vi "CustomGaugeFacade.vi"(0 "Data In":T4, 2 "Display State In":T2, 3 "Container State":T3) -> (6 "Data Out":T4, 7 "Display State Out":T2, 8 "Action":T1)   [LabVIEW 2012, in "CustomGauge.xctl"]
uses:
  CustomGauge.xctl
  CustomGaugeData.ctl
  <vilib>/_xctls/Container State.ctl
  CustomGaugeState.ctl
  <vilib>/_xctls/Action.ctl
  <vilib>/_xctls/XControlSupport.lvlib
panel:
  in  "Gauge":dbl(knob) scale=0.0..10.0
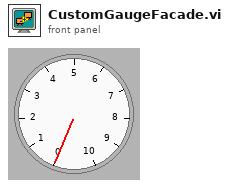
[diagram p1: front panel]
types:
  T1 = typedef "XControlSupport.lvlib/Action.ctl" = cluster{"Data Changed?":bool, "State Changed?":bool, "Action Name":string}
  T2 = typedef "CustomGauge.xctl/CustomGaugeState.ctl" = cluster{"Shared Variable Control":refnum<k21>}
  T3 = typedef "XControlSupport.lvlib/Container State.ctl" = cluster{"Indicator?":bool, "Run Mode?":bool, " Refnum":refnum<vi>}
  T4 = typedef "CustomGauge.xctl/CustomGaugeData.ctl" = dbl
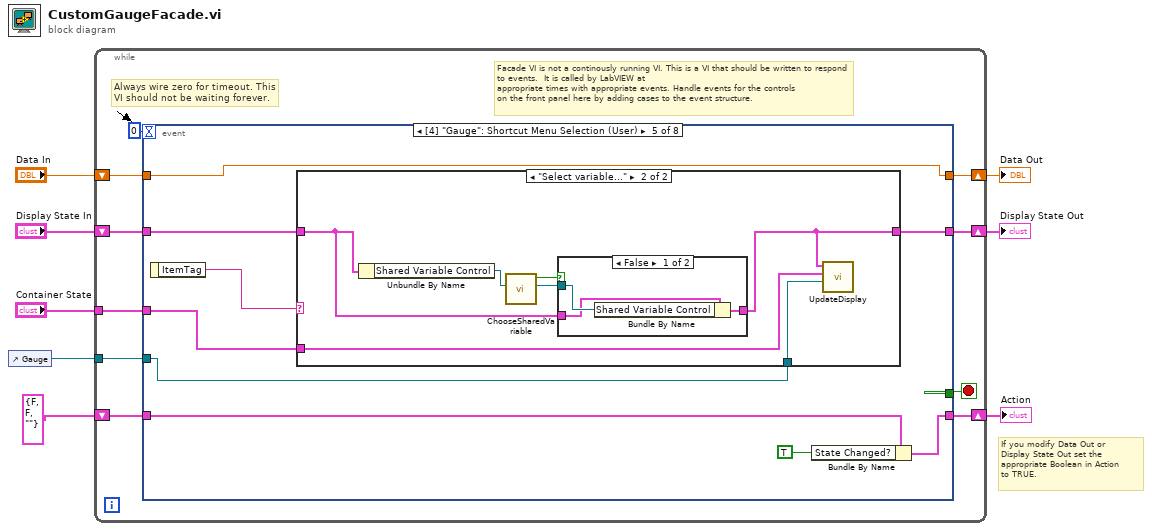
[diagram p0: block diagram]
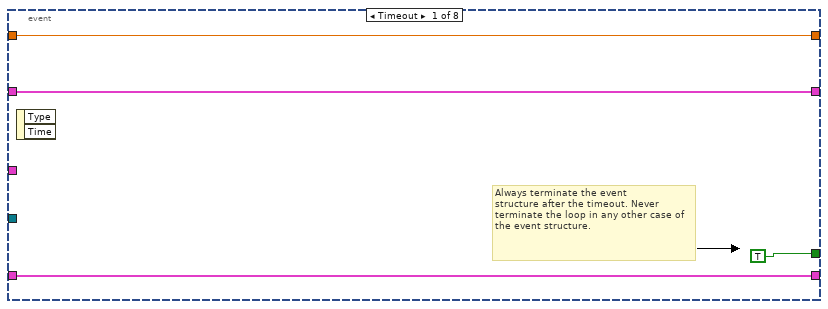
[diagram p2: hidden frame]
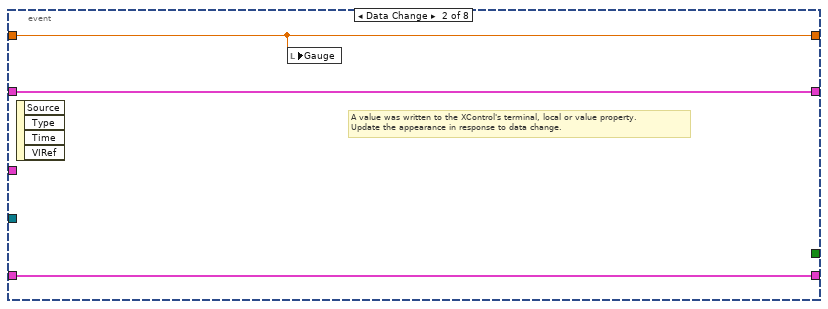
[diagram p3: hidden frame]
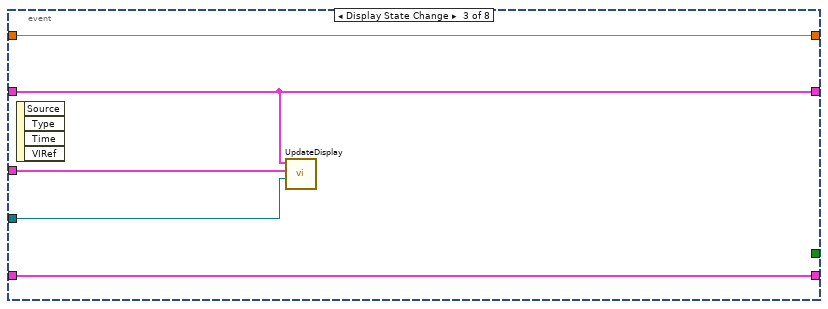
[diagram p4: hidden frame]
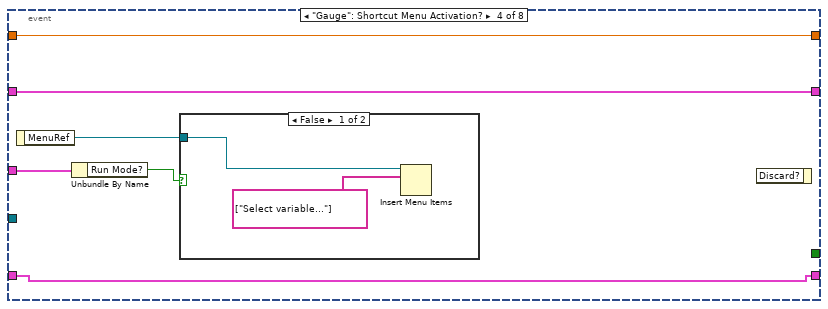
[diagram p5: hidden frame]
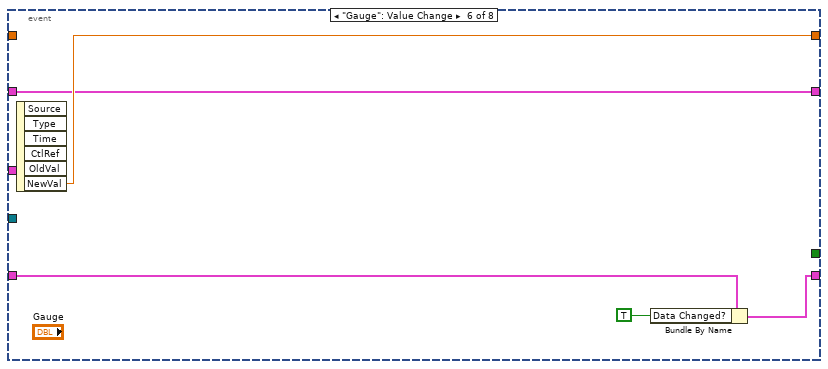
[diagram p9: hidden frame]
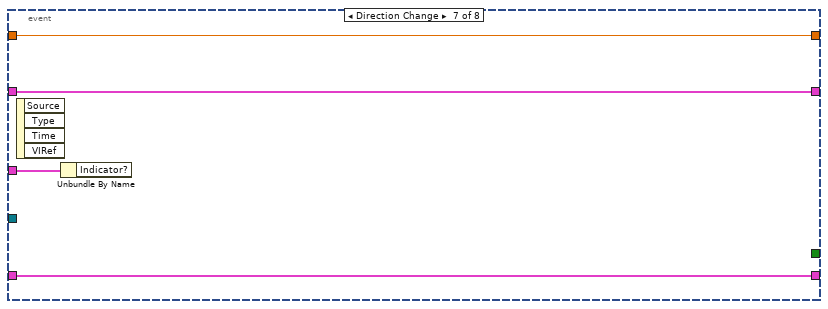
[diagram p10: hidden frame]
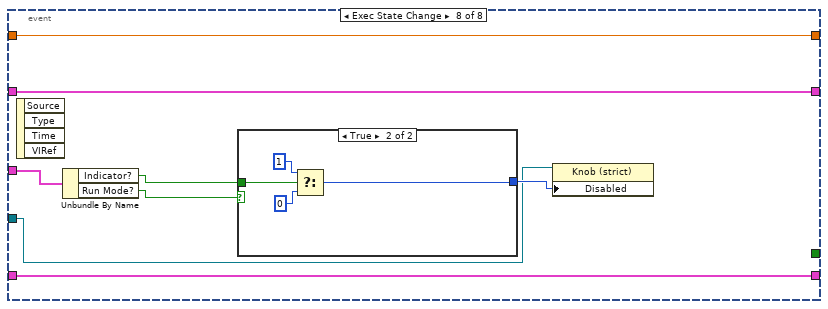
[diagram p11: hidden frame]
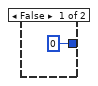
[diagram p12: hidden frame]
diagram:
  # "If you modify Data Out or\nDisplay State Out set the\nappropriate Boolean in Action\nto TRUE."
  n1 = control-ref of="Gauge"() -> (w1:refnum<vi>)
  n2 = while {
    shift-right: [w17] -> w5
    shift-left: "Display State In" -> [w18]
    tunnel: "Container State" -> [w14]
    shift-right: [w12] -> w8
    shift-left: "Data In" -> [w13]
    shift-right: [w10] -> w3
    shift-left: T1 {"Data Changed?"=FALSE, "State Changed?"=FALSE, "Action Name"=""} ("Action") -> [w11]
    tunnel: w1 -> [w9]
    stop <- w16 stop-if-true
    # "Facade VI is not a continously running VI. This is a VI that should be written to respond to events.  It is called by LabVIEW at\nappropriate times with appropriate events. Handle events for the controls\non the front panel here by adding cases to the event structure."
    # "Always wire zero for timeout. This\nVI should not be waiting forever."
    n3 = event shown="[4] \"Gauge\": Shortcut Menu Selection (User)" {
      selector: _ -> [_ _ _ _ _ _ _ _]
      dyn-events: _ -> [_ _ _ _ _ _ _ _]
      timeout: 0 -> [_ _ _ _ _ _ _ _]
      tunnel: w18 -> [w20 w25 w28 w35 w46 w63 w67 w75]
      tunnel: [w20 w25 w28 w35 w45 w63 w67 w75] -> w17
      tunnel: [TRUE _ _ _ _ _ _ _] -> w16
      tunnel: w14 -> [_ _ w27 w32 w40 _ w68 w76]
      tunnel: w13 -> [w19 w23 w30 w34 w44 _ w66 w74]
      tunnel: [w19 w23 w30 w34 w44 w64 w66 w74] -> w12
      tunnel: [w21 w24 w29 w33 w43 w62 w65 w73] -> w10
      tunnel: w11 -> [w21 w24 w29 w33 w42 w61 w65 w73]
      tunnel: w9 -> [_ _ w26 _ w39 _ _ w69]
      event Timeout {
        # "Always terminate the event\nstructure after the timeout. Never terminate the loop in any other case of the event structure."
        n4 = event-data() -> ()  [unwired: 1 in, 2 out]
      }
      event Data Change {
        # "A value was written to the XControl's terminal, local or value property.\nUpdate the appearance in response to data change."
        n5 = event-data() -> ()  [unwired: 1 in, 4 out]
        n6 = local write "Gauge"(w23) -> ()
      }
      event Display State Change {
        n7 = event-data() -> ()  [unwired: 1 in, 4 out]
        n8 = call "UpdateDisplay.vi"("Gauge"=w26, "Container State"=w27, "Display State In"=w28) -> ()  [unwired: 7 in, 1 out]
      }
      event "Gauge": Shortcut Menu Activation? {
        n9 = event-data() -> ("MenuRef"=w36:refnum<k9>)  [unwired: 1 in]
        n10 = Unbundle By Name(w32) -> ("Run Mode?"=w31:bool)
        n11 = case shown="False" w31 {
          tunnel: w36 -> [w38 _]
          frame False {
            n12 = Insert Menu Items(8:string[] ["Select variable..."] ("item names"), 9:w38) -> ()  [unwired: 4 in, 3 out]
          }
          frame True {
          }
        }
        n13 = event-data() -> ()  [unwired: 2 in, 1 out]
      }
      event "Gauge": Shortcut Menu Selection (User) {
        n14 = event-data() -> ("ItemTag"=w47:string)  [unwired: 1 in]
        n15 = case shown="\"Select variable...\"" w47 {
          tunnel: w46 -> [w48 w52]
          tunnel: [w48 w51] -> w45
          tunnel: w40 -> [_ w50]
          tunnel: w39 -> [_ w49]
          frame Default {
          }
          frame "Select variable..." {
            n16 = Unbundle By Name(w52) -> ("Shared Variable Control"=w53:refnum<k21>)
            n17 = call "ChooseSharedVariable.vi"("Select published shared variable to bind to..."=w53) -> ("Shared Variable"=w54:refnum<k21>, "Cancelled?"=w55:bool)  [unwired: 9 in]
            n18 = case shown="False" w55 {
              tunnel: w54 -> [w58 _]
              tunnel: [w57 w59] -> w51
              tunnel: w52 -> [w56 w59]
              frame False {
                n19 = Bundle By Name(cluster=w56, "Shared Variable Control"=w58) -> (w57:T2)
              }
              frame True {
              }
            }
            n20 = call "UpdateDisplay.vi"("Gauge"=w49, "Container State"=w50, "Display State In"=w51) -> ()  [unwired: 7 in, 1 out]
          }
        }
        n21 = Bundle By Name(cluster=w42, "State Changed?"=TRUE) -> (w43:T1)
      }
      event "Gauge": Value Change {
        n22 = event-data() -> ("NewVal"=w64:dbl)  [unwired: 1 in, 5 out]
        n23 = Bundle By Name(cluster=w61, "Data Changed?"=TRUE) -> (w62:T1)
      }
      event Direction Change {
        n24 = event-data() -> ()  [unwired: 1 in, 4 out]
        n25 = Unbundle By Name(w68) -> ()  [unwired: 1 out]
      }
      event Exec State Change {
        n26 = event-data() -> ()  [unwired: 1 in, 4 out]
        n27 = Unbundle By Name(w76) -> ("Indicator?"=w71:bool, "Run Mode?"=w70:bool)
        n28 = case shown="True" w70 {
          tunnel: [u8 0 ("Disabled") w79] -> w72
          tunnel: w71 -> [_ w78]
          frame False {
          }
          frame True {
            n29 = Select(t=u8 1 ("Disabled"), s=w78, f=u8 0 ("Disabled")) -> (s? t:f=w79:u8)
          }
        }
        n30 = property class="Knob (strict)"(reference=w69, "Disabled"=w72) -> ()  [unwired: 1 in, 2 out]
      }
    }
  }
  "Display State Out" <- w5
  "Data Out" <- w8
  "Action" <- w3
